vi "Read_DBL_from_Excel.vi"(8 "error in (no error)":errorcluster, 9 "Colunm":i32, 10 "row":i32, 11 "NI_report in":refnum<class "NI_report.lvclass">) -> (0 "error out":errorcluster, 2 "data":dbl, 3 "NI_report Out":refnum<class "NI_report.lvclass">)   [LabVIEW 2015]
uses:
  <vilib>/Utility/NIReport.llb/NI_report.lvclass
  <vilib>/addons/_office/excel.llb/Excel Get Data (dbl).vi
  <vilib>/addons/_office/NI_ReportGenerationToolkit.lvlib
  <vilib>/Utility/NIReport.llb/Excel/NI_Excel.lvclass
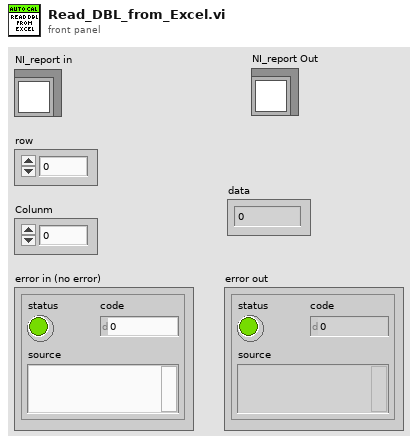
[diagram p1: front panel]
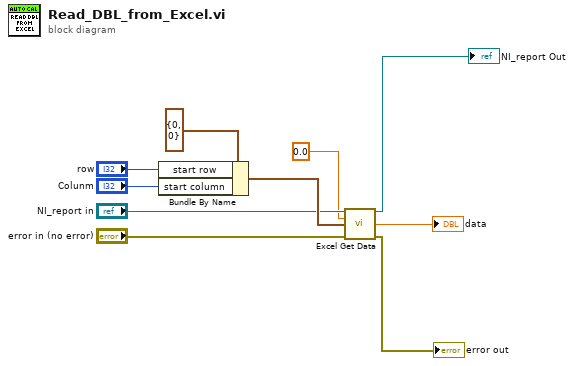
[diagram p0: block diagram]
diagram:
  n1 = Bundle By Name(cluster=cluster{"start row":i32, "start column":i32} {"start row"=0, "start column"=0} ("start (0, 0)"), "start row"="row", "start column"="Colunm") -> (w9:cluster{"start row":i32, "start column":i32})
  n2 = call-poly <vilib>:"Excel Get Data.vi"("report in"="NI_report in", "data type"=0.0, "start (0, 0)"=w9, "error in (no error)"="error in (no error)") -> ("report out"=→"NI_report Out":refnum<class "NI_report.lvclass">, "data"=→"data":dbl, "error out"=→"error out":errorcluster)  [unwired: 9 in]
